vi "Configure Serial Bus (A429 - Trigger).vi"(0 "VISA resource name":refnum<visa-resource-name>, 1 "Data Pattern (XXXXXXXXXXXXXXXXXXX)":string="XXXXXXXXXXXXXXXXXXX", 2 "SSM Pattern (XX)":string="XX", 3 "Higher Threshold (1)":i32=1, 5 "Serial Bus Name (1: Serial Bus 1)":i32(ring)=1 items=["Serial Bus 1"=1, "Serial Bus 2"=2], 7 "Trigger Type (0: Wstart)":i32(ring) items=["Word Start", "Word Stop", "Label", "Label Bits", "Label Range", "Parity Error", "Word Error", "Gap Error", "Word or Gap Errors", "All Errors", "Any Bits", "Any One Bits", "Any Zero Bits"], 9 "Trigger Label (-1)":i32=-1, 11 "error in (no error)":errorcluster, 12 "SDI Pattern (XX)":string="XX", 13 "Lower Threshold (0)":i32) -> (4 "VISA resource name out":refnum<visa-resource-name>, 15 "error out":errorcluster)   [LabVIEW 2015, in "Agilent 2000 3000 X-Series.lvlib"]
doc: "Configures the trigger settings of ARINC 429 bus.\n\nNote:\nThis VI is not supported by EDUX1052A, EDUX1052G, DSOX1202A, DSOX1202G, DSOX1204A, DSOX1204G models"
uses:
  Agilent 2000 3000 X-Series.lvlib
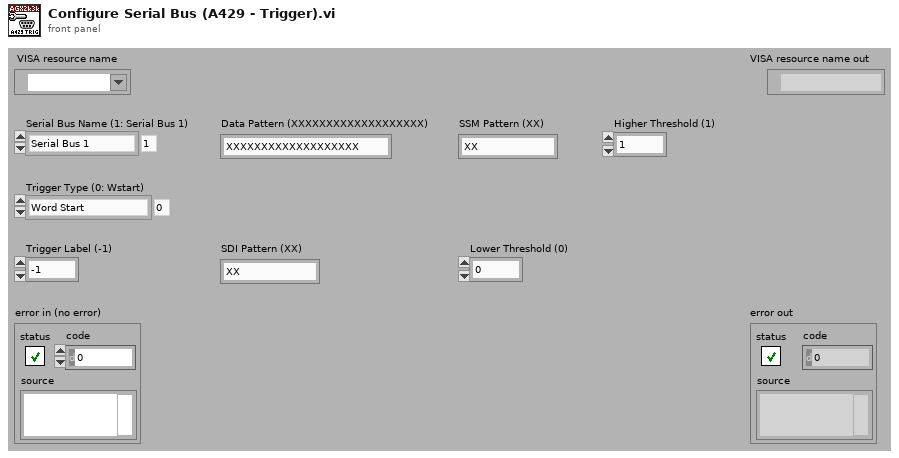
[diagram p1: front panel]
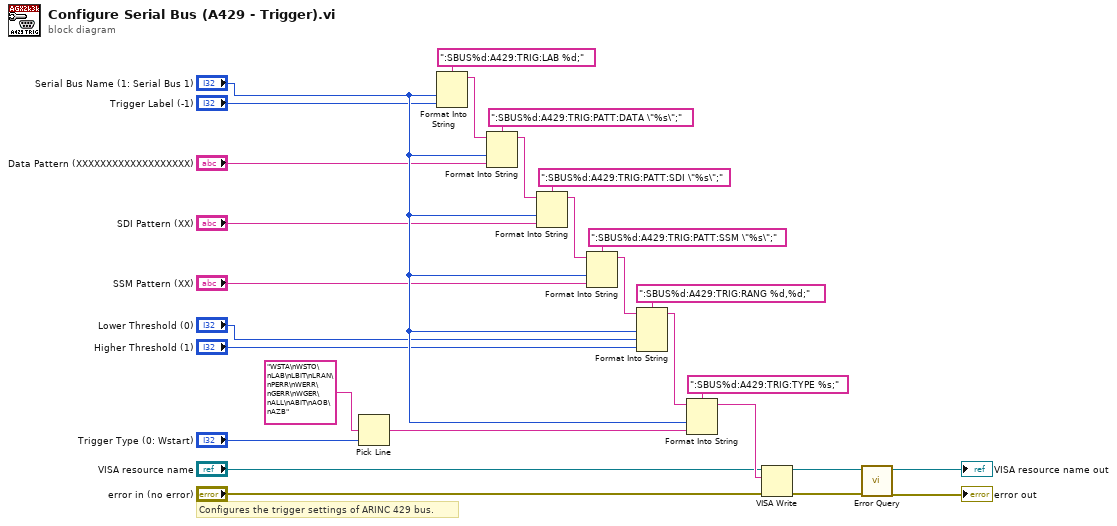
[diagram p0: block diagram]
diagram:
  # "Configures the trigger settings of ARINC 429 bus."
  n1 = Pick Line(multi-line string="WSTA\nWSTO\nLAB\nLBIT\nLRAN\nPERR\nWERR\nGERR\nWGER\nALL\nABIT\nAOB\nAZB", line index="Trigger Type (0: Wstart)") -> (output string=w8:string)  [unwired: 1 out]
  n2 = Format Into String(format string=":SBUS%d:A429:TRIG:LAB %d;", "Serial Bus Name (1: Serial Bus 1)", "Trigger Label (-1)") -> (resulting string=w25:string)  [unwired: 2 in, 1 out]
  n3 = Format Into String(format string=":SBUS%d:A429:TRIG:PATT:DATA \"%s\";", initial string=w25, "Serial Bus Name (1: Serial Bus 1)", "Data Pattern (XXXXXXXXXXXXXXXXXXX)") -> (resulting string=w22:string)  [unwired: 1 in, 1 out]
  n4 = Format Into String(format string=":SBUS%d:A429:TRIG:PATT:SDI \"%s\";", initial string=w22, "Serial Bus Name (1: Serial Bus 1)", "SDI Pattern (XX)") -> (resulting string=w19:string)  [unwired: 1 in, 1 out]
  n5 = Format Into String(format string=":SBUS%d:A429:TRIG:PATT:SSM \"%s\";", initial string=w19, "Serial Bus Name (1: Serial Bus 1)", "SSM Pattern (XX)") -> (resulting string=w16:string)  [unwired: 1 in, 1 out]
  n6 = Format Into String(format string=":SBUS%d:A429:TRIG:RANG %d,%d;", initial string=w16, "Serial Bus Name (1: Serial Bus 1)", "Lower Threshold (0)", "Higher Threshold (1)") -> (resulting string=w10:string)  [unwired: 1 in, 1 out]
  n7 = Format Into String(format string=":SBUS%d:A429:TRIG:TYPE %s;", initial string=w10, "Serial Bus Name (1: Serial Bus 1)", w8) -> (resulting string=w7:string)  [unwired: 1 in, 1 out]
  n8 = VISA Write(VISA resource name="VISA resource name", write buffer=w7, error in (no error)="error in (no error)") -> (VISA resource name out=w4:refnum<visa-resource-name>, error out=w3:errorcluster)  [unwired: 1 out]
  n9 = call "Error Query.vi"("error in (no error)"=w3, "VISA resource name"=w4) -> ("error out"=→"error out":errorcluster, "VISA resource name out"=→"VISA resource name out":refnum<visa-resource-name>)  [unwired: 8 out]
